vi "Test_RequestSynchronousDatum_DoubleX_NotPublished_TimeoutError.vi"(8 "error in (no error)":errorcluster, 11 "TestCase in":refnum<class "TestRequestSynchronousData.lvclass">) -> (0 "error out":errorcluster, 3 "TestCase out":refnum<class "TestRequestSynchronousData.lvclass">)   [LabVIEW 2020, in "TestRequestSynchronousData.lvclass"]
uses:
  TestRequestSynchronousData.lvclass
  TestRequestSynchronousData.lvclass/TestRequestSynchronousData.ctl
  24bf8875-c008-4f22-9bfa-88e42476d167.vi
  Source/IModel/IModel/IModel.lvclass
  <vilib>/ActorFramework/Actor/Actor.lvclass
  Source/Mediator/Mediator/Mediator.lvclass
  <vilib>/ActorFramework/Stop Msg/Stop Msg.lvclass
  modules/composed-event-logger/Source/String Control Sink/String Control Sink.lvclass
  f7bee35d-b044-4098-91af-55574313c386.vi
  modules/composed-event-logger/Source/Composed Log/LoggerReference/LoggerReference.lvclass
  11850773-0e08-463b-84b0-7f64b956e994.vi
  Source/RootModel/RootModel/RootModel.lvclass
  C:/Git/mva-core/Source/IModel/IModel/IModel.lvclass
  C:/Git/mva-core/Source/IObserver/IObserver/IObserver.lvclass
  C:/Program Files (x86)/National Instruments/LabVIEW 2020/vi.lib/ActorFramework/Actor/Actor.lvclass
  C:/Git/mva-core/Source/RootModel/RootModel/RootModel.lvclass
  Doubles/ModelSynchronouslyRequestsDoubleFloat/ModelSynchronouslyRequestsDoubleFloat.lvclass
  C:/Git/mva-core/Test/Doubles/ModelSynchronouslyRequestsDoubleFloat/ModelSynchronouslyRequestsDoubleFloat.lvclass
panel:
  out "Request Result":T1
  out "Log":string
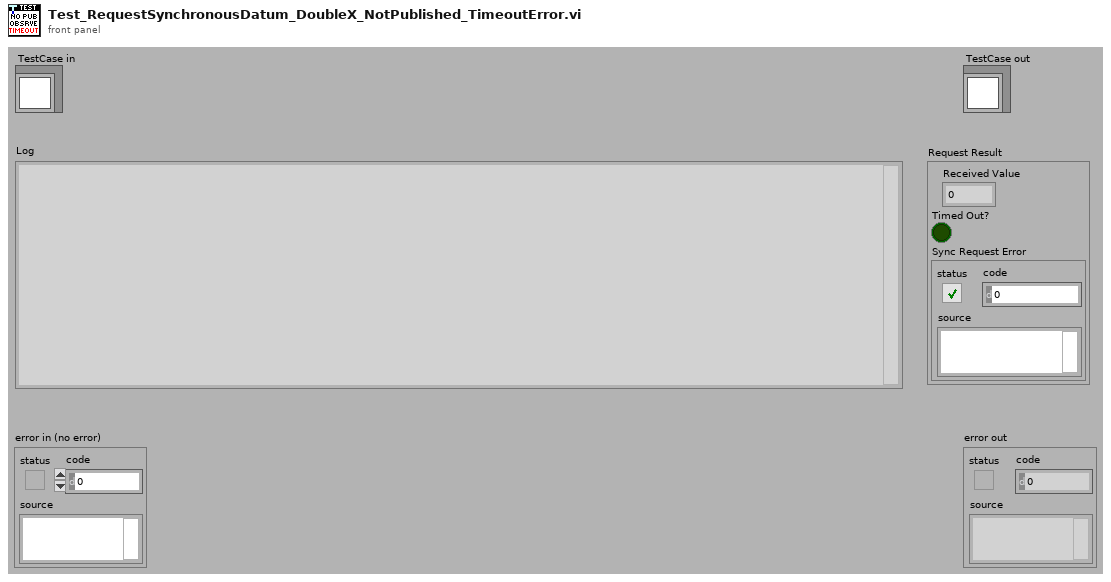
[diagram p1: front panel]
types:
  T1 = cluster{"Received Value":dbl, "Timed Out?":bool, "Sync Request Error":errorcluster}
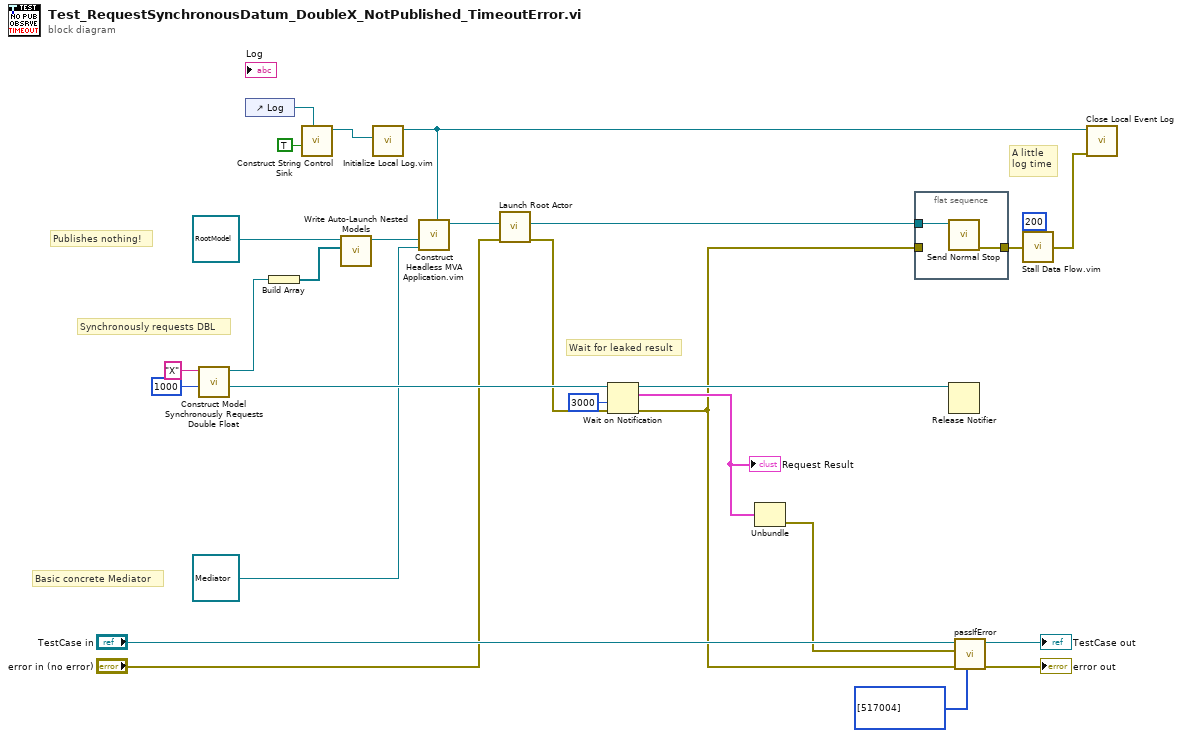
[diagram p0: block diagram]
diagram:
  # "A little\nlog time"
  # "Wait for leaked result"
  # "Basic concrete Mediator"
  # "Synchronously requests DBL"
  # "Publishes nothing!"
  n1 = call "Construct Model Synchronously Requests Double Float.vi"("DBL Request Timeout (2000)"=1000, "DBL Name"="X") -> ("Result Notifier"=w28:refnum<notifier>, "ModelSynchronouslyRequestsDoubleFloat Out"=w8:refnum<class "ModelSynchronouslyRequestsDoubleFloat.lvclass">)  [unwired: 8 in]
  n2 = control-ref of="Log"() -> (w15:refnum<vi>)
  n3 = Build Array(w8) -> (w23:refnum<class "ModelSynchronouslyRequestsDoubleFloat.lvclass">[])
  n4 = call "Construct String Control Sink.vi"("Str Refnum"=w15, "AutoScroll?(F)"=TRUE) -> ("String Control Sink out"=w14:refnum<class "String Control Sink.lvclass">)  [unwired: 9 in]
  n5 = call "Write Auto-Launch Nested Models.vi"("Auto-Launch Nested Models"=w23, "IModel In"=refnum<class "RootModel.lvclass"> refnum ("RootModelPublishesDoubleFloatX.lvclass")) -> ("IModel Out"=w22:refnum<class "RootModel.lvclass">)  [unwired: 9 in]
  n6 = call "Initialize Local Log.vim"("Startup Sink(s)"=w14) -> ("Log Instance Reference"=w12:refnum<class "LoggerReference.lvclass">)  [unwired: 8 in, 2 out]
  n7 = call "Construct Headless MVA Application.vim"("Parent Log Reference"=w12, "Mediator Type"=refnum<class "Mediator.lvclass"> refnum ("Mediator.lvlib:Mediator.lvclass"), "RootModel in"=w22) -> ("RootModel out"=w21:refnum<class "RootModel.lvclass">)  [unwired: 8 in]
  n8 = call <vilib>:"Launch Root Actor.vi"("error in (no error)"="error in (no error)", "Actor"=w21) -> ("error out"=w2:errorcluster, "Actor's Enqueuer"=w17:refnum<class "Message Enqueuer.lvclass">)  [unwired: 8 in]
  n9 = Wait on Notification(notifier=w28, timeout in ms (-1)=3000, error in (no error)=w2) -> (notifier out=w20:refnum<notifier>, notification=w6:T1, error out=w1:errorcluster)  [unwired: 1 in, 1 out]
  "Request Result" <- w6
  n10 = Unbundle(w6) -> ("Sync Request Error"=w4:errorcluster)  [unwired: 2 out]
  n11 = flat-sequence {
    tunnel: w17 -> [w30]
    tunnel: [w29] -> w11
    tunnel: w1 -> [_]
    frame #0 {
      n12 = call <vilib>:"Send Normal Stop.vi"("Message Enqueuer"=w30) -> ("error out"=w29:errorcluster)  [unwired: 10 in]
    }
  }
  n13 = Release Notifier(notifier=w20) -> ()  [unwired: 2 in, 3 out]
  n14 = call-dynamic "passIfError.vi"("passing error codes (default = any error code)"=i32[] [517004], "error in (no error)"=w1, "error"=w4, "TestCase in"="TestCase in") -> ("error out"=→"error out":errorcluster, "TestCase out"=→"TestCase out":refnum<class "TestRequestSynchronousData.lvclass">)  [unwired: 6 in]
  n15 = call "Stall Data Flow.vim"("value in"=w11, "milliseconds to wait"=u32 200) -> ("value out"=w10:errorcluster)  [unwired: 1 out]
  n16 = call "Close Local Event Log.vi"("error in (no error)"=w10, "Log Instance"=w12) -> ()  [unwired: 9 in, 1 out]
